vi "Ensure File Exists.vi"(8 "error in (no error)":errorcluster, 11 "Approved":path) -> (0 "error out":errorcluster, 3 "File Path":path)   [LabVIEW 2020, in "Approval Tests.lvlib"]
uses:
  Report With Beyord Compare/Report With Beyond Compare.lvclass/Report With Beyond Compare.ctl
  Approval Tests.lvlib
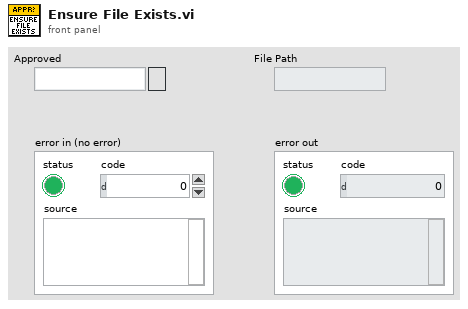
[diagram p1: front panel]
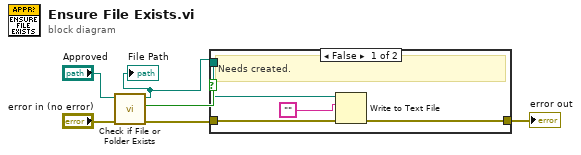
[diagram p0: block diagram]
diagram:
  n1 = call <vilib>:"Check if File or Folder Exists.vi"("error in (no error)"="error in (no error)", "path"="Approved") -> ("error out"=w3:errorcluster, "file or folder exists?"=w4:bool, "dup path"=w1:path)  [unwired: 7 in]
  "File Path" <- w1
  n2 = case shown="False" w4 {
    tunnel: w3 -> [w10 w11]
    tunnel: [w9 w11] -> w2
    tunnel: w1 -> [w8 _]
    frame False {
      # "Needs created."
      n3 = Write to Text File(file (use dialog)=w8, text="", error in=w10) -> (error out=w9:errorcluster)  [unwired: 1 in, 2 out]
    }
    frame True {
      # "Does exist"
    }
  }
  "error out" <- w2
